vi "Example Before.vi"() -> ()   [LabVIEW 2019, in "LSS.lvlib"]
doc: "This example demonstrates how a user can save time developing user interfaces using LSS by showing how a simple application that uses property nodes to change style at runtime can be transitioned to using LSS. The \"Example Before.vi\" contains one way the code could have been written using arrays of property nodes. The \"Example After.vi\" is a functionally equivalent piece of code that uses LSS instead. Example After.vi uses no property nodes or manually created references to perform the exact same operations."
uses:
  LSS.lvlib
  SubVIs/Example SubVIs/Before SubVIs/Themes.ctl
  SubVIs/Example SubVIs/Before UI References.ctl
panel:
  out "mode":T1
  in  "Dialog":bool
  in  "Normal":bool
  in  "Small":bool
  in  "Slide 2":dbl(slide) scale=0.0..10.0
  out "Stat2":dbl
  out "Stat1":dbl
  out "Pressure":dbl
  out "Time":dbl
  in  "Slide":dbl(slide) scale=0.0..10.0
  in  "THEME2":bool
  in  "THEME1":bool
  in  "COMPANY":bool
  out "Mars":picture
  in  "SPACE":bool
  out "Map":picture
  out "Vortex":picture
  out "Chart 3":dbl(graph)
  out "Chart 2":dbl(graph)
  out "Chart1":dbl(graph)
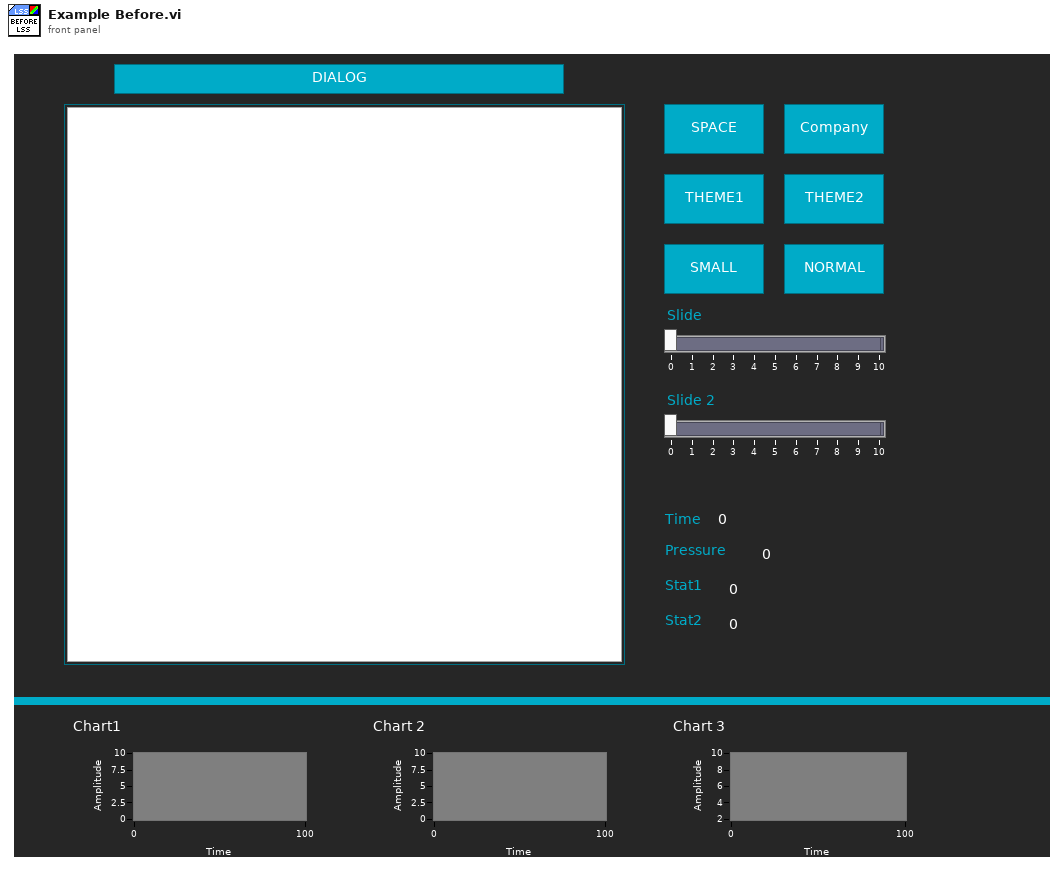
[diagram p1: front panel]
types:
  T1 = typedef "LSS.lvlib/Themes.ctl" = enum16{"SPACE", "COMPANY", "THEME1", "THEME2"}
  T2 = typedef "LSS.lvlib/Before UI References.ctl" = cluster{"Panes":refnum<vi>[], "Splitter":refnum<vi>, "Mars Picture":refnum<vi>, "Buttons":refnum<vi>[], "Numerics":refnum<vi>[], "Graphs":refnum<vi>[], "Slides":refnum<vi>[], "This VI":refnum<vi>, "Vortex":refnum<vi>, "Map":refnum<vi>}
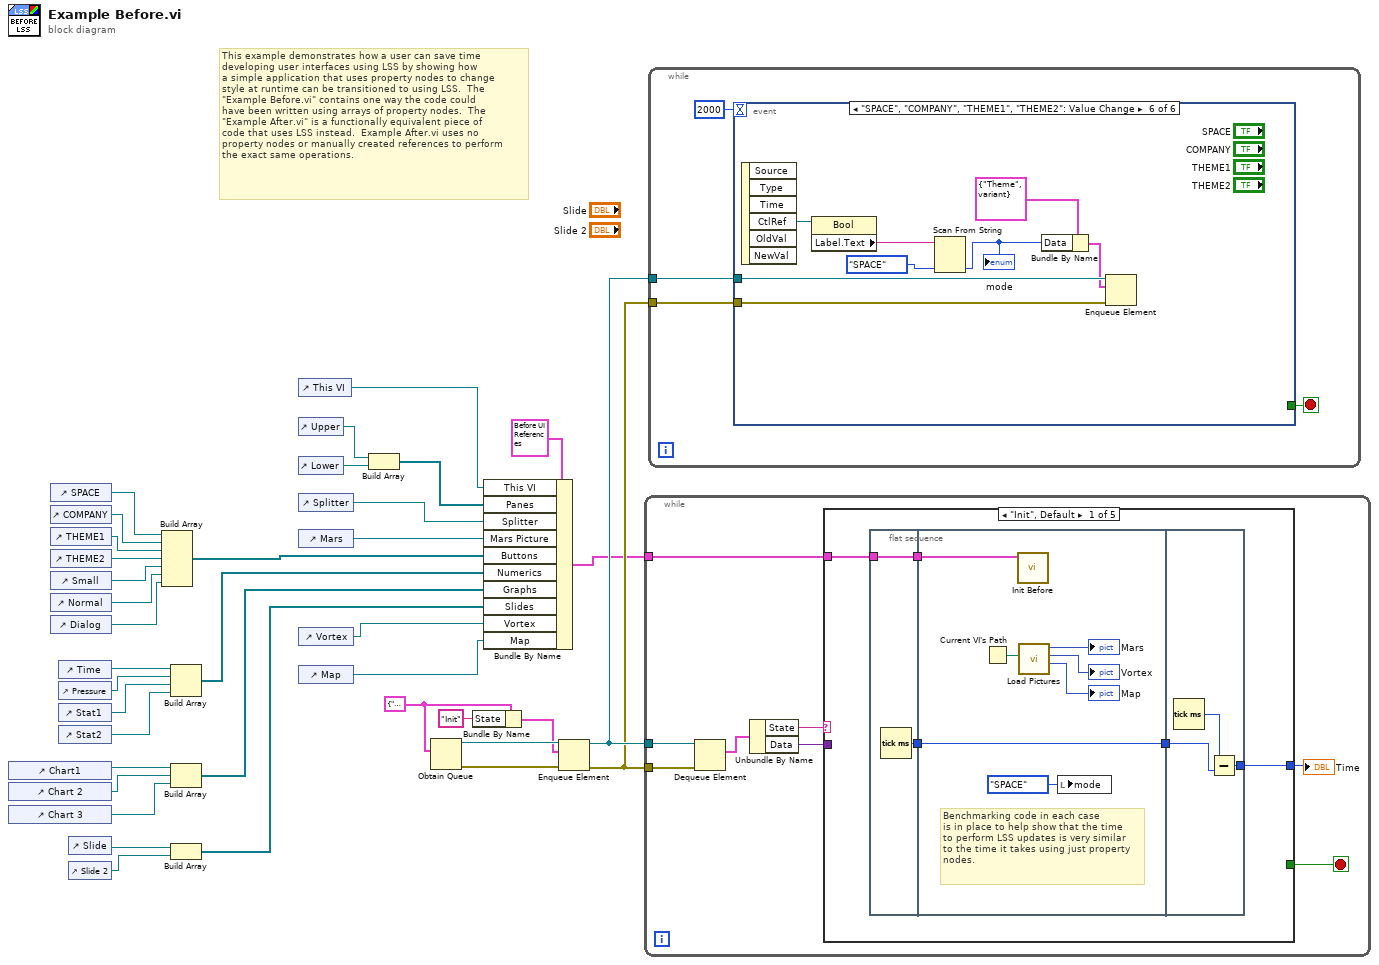
[diagram p0: block diagram]
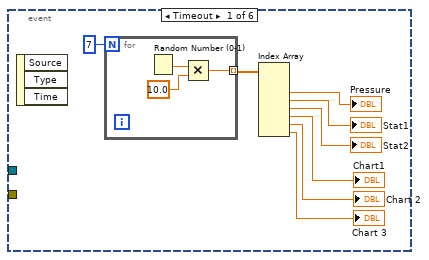
[diagram p2: hidden frame]
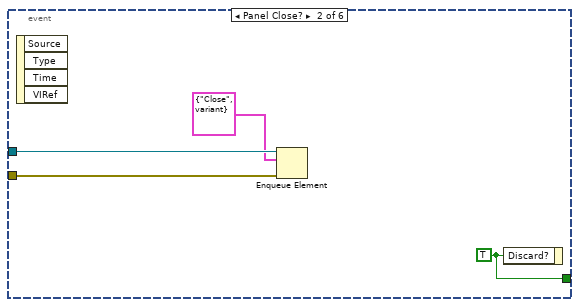
[diagram p3: hidden frame]
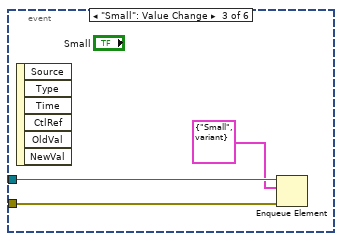
[diagram p4: hidden frame]
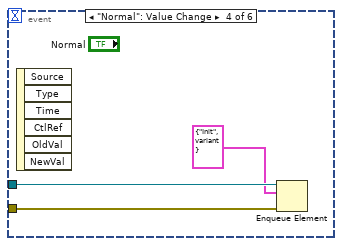
[diagram p5: hidden frame]
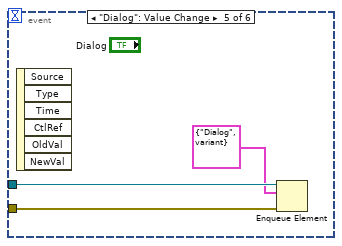
[diagram p6: hidden frame]
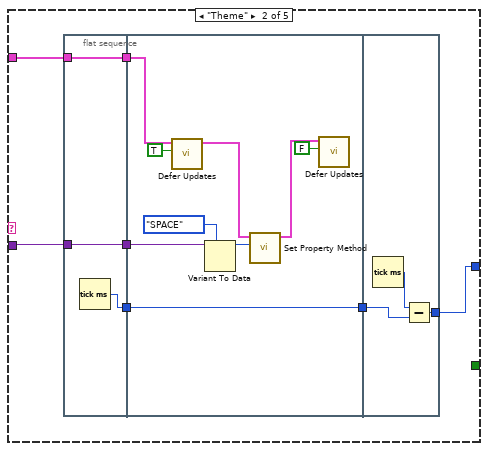
[diagram p7: hidden frame]
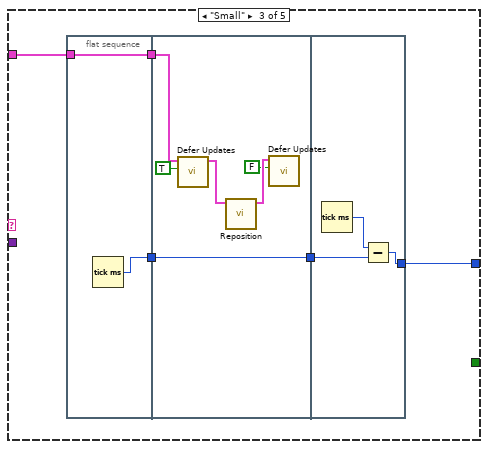
[diagram p8: hidden frame]
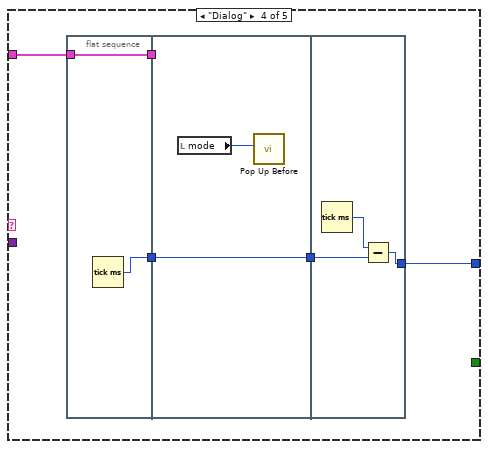
[diagram p9: hidden frame]
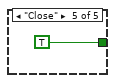
[diagram p10: hidden frame]
diagram:
  w35 = cluster{"State":string, "Data":variant} {"State"="", "Data"=variant}
  # "This example demonstrates how a user can save time\ndeveloping user interfaces using LSS by showing how\na simple application that uses property nodes to change\nstyle at runtime can be transitioned to using LSS.  The\n\"Example Before.vi\" contains one way the code could\nhave been written using arrays of property nodes.  The\n\"Example After.vi\" is a functionally equivalent piece of\ncode that uses LSS instead.  Example After.vi uses no\nproperty nodes or manually created references to perform\nthe exact same operations."
  n1 = control-ref of="Chart1"() -> (w14:refnum<vi>)
  n2 = control-ref of="Chart 2"() -> (w13:refnum<vi>)
  n3 = control-ref of="Chart 3"() -> (w12:refnum<vi>)
  n4 = control-ref of="SPACE"() -> (w20:refnum<vi>)
  n5 = control-ref of="COMPANY"() -> (w21:refnum<vi>)
  n6 = control-ref of="THEME1"() -> (w22:refnum<vi>)
  n7 = control-ref of="THEME2"() -> (w23:refnum<vi>)
  n8 = control-ref of="Small"() -> (w6:refnum<vi>)
  n9 = control-ref of="Normal"() -> (w5:refnum<vi>)
  n10 = control-ref of="Dialog"() -> (w3:refnum<vi>)
  n11 = control-ref of="Time"() -> (w18:refnum<vi>)
  n12 = control-ref of="Pressure"() -> (w17:refnum<vi>)
  n13 = control-ref of="Stat1"() -> (w16:refnum<vi>)
  n14 = control-ref of="Stat2"() -> (w15:refnum<vi>)
  n15 = control-ref of="Slide"() -> (w11:refnum<vi>)
  n16 = control-ref of="Slide 2"() -> (w10:refnum<vi>)
  n17 = Build Array(w20, w21, w22, w23, w6, w5, w3) -> (w19:refnum<vi>[])
  n18 = Build Array(w18, w17, w16, w15) -> (w9:refnum<vi>[])
  n19 = Build Array(w14, w13, w12) -> (w8:refnum<vi>[])
  n20 = Build Array(w11, w10) -> (w7:refnum<vi>[])
  n21 = control-ref of="This VI"() -> (w4:refnum<vi>)
  n22 = control-ref of="Upper"() -> (w30:refnum<vi>)
  n23 = control-ref of="Lower"() -> (w29:refnum<vi>)
  n24 = control-ref of="Splitter"() -> (w26:refnum<vi>)
  n25 = control-ref of="Mars"() -> (w25:refnum<vi>)
  n26 = control-ref of="Vortex"() -> (w2:refnum<vi>)
  n27 = control-ref of="Map"() -> (w1:refnum<vi>)
  n28 = Build Array(w30, w29) -> (w27:refnum<vi>[])
  n29 = Obtain Queue(element data type=w35) -> (queue out=w37:refnum<queue>, error out=w36:errorcluster)  [unwired: 4 in, 1 out]
  n30 = Bundle By Name(cluster=w35, "State"="Init") -> (w33:cluster{"State":string, "Data":variant})
  n31 = Bundle By Name(cluster=T2 {"Panes"=[], "Splitter"=refnum, "Mars Picture"=refnum, "Buttons"=[], "Numerics"=[], "Graphs"=[], "Slides"=[], "This VI"=refnum, "Vortex"=refnum, "Map"=refnum}, "This VI"=w4, "Panes"=w27, "Splitter"=w26, "Mars Picture"=w25, "Buttons"=w19, "Numerics"=w9, "Graphs"=w8, "Slides"=w7, "Vortex"=w2, "Map"=w1) -> (w24:T2)
  n32 = Enqueue Element(queue=w37, element=w33, error in (no error)=w36) -> (queue out=w32:refnum<queue>, error out=w31:errorcluster)  [unwired: 1 in, 1 out]
  n33 = while {
    tunnel: w32 -> [w45]
    tunnel: w31 -> [w44]
    tunnel: w24 -> [w39]
    stop <- w40 stop-if-true
    n34 = Dequeue Element(queue=w45, error in (no error)=w44) -> (element=w43:cluster{"State":string, "Data":variant})  [unwired: 1 in, 3 out]
    n35 = Unbundle By Name(w43) -> ("State"=w42:string, "Data"=w41:variant)
    n36 = case shown="\"Init\", Default" w42 {
      tunnel: w41 -> [_ w69 _ _ _]
      tunnel: [_ _ _ _ TRUE] -> w40
      tunnel: w39 -> [w50 w68 w89 w105 _]
      tunnel: [w46 w63 w85 w101 _] -> w38
      frame "Init", Default {
        n37 = flat-sequence {
          tunnel: w50 -> [w52]
          tunnel: [w52] -> w49
          tunnel: [w51] -> w48
          tunnel: w49 -> [w58]
          tunnel: w48 -> [w55]
          tunnel: [w55] -> w47
          tunnel: w47 -> [w62]
          tunnel: [w60] -> w46
          frame #0 {
            n38 = Tick Count (ms)() -> (millisecond timer value=w51:u32)
          }
          frame #1 {
            # "Benchmarking code in each case\nis in place to help show that the time\nto perform LSS updates is very similar\nto the time it takes using just property\nnodes."
            n39 = Current VI's Path() -> (path=w53:path)
            n40 = call "Init Before.vi"("Cluster"=w58) -> ()  [unwired: 11 in]
            n41 = call "Load Pictures.vi"("Application Directory"=w53) -> ("Map"=→"Map":picture, "Vortex"=→"Vortex":picture, "Mars"=→"Mars":picture)  [unwired: 8 in]
            n42 = local write "mode"(Themes."SPACE" ("mode")) -> ()
          }
          frame #2 {
            n43 = Tick Count (ms)() -> (millisecond timer value=w61:u32)
            n44 = Subtract(x=w61, y=w62) -> (x-y=w60:u32)
          }
        }
      }
      frame "Theme" {
        n45 = flat-sequence {
          tunnel: w68 -> [w71]
          tunnel: w69 -> [w72]
          tunnel: [w72] -> w67
          tunnel: [w71] -> w66
          tunnel: [w70] -> w64
          tunnel: w67 -> [w81]
          tunnel: w66 -> [w77]
          tunnel: [w78] -> w65
          tunnel: w64 -> [w78]
          tunnel: w65 -> [w83]
          tunnel: [w82] -> w63
          frame #0 {
            n46 = Tick Count (ms)() -> (millisecond timer value=w70:u32)
          }
          frame #1 {
            n47 = call "Defer Updates.vi"("Defer Panel Updates"=TRUE, "Cluster"=w77) -> ("Cluster Out"=w75:T2)  [unwired: 8 in, 1 out]
            n48 = Variant To Data(type=Themes."SPACE" ("Theme Choice"), Variant=w81) -> (data=w79:T1)  [unwired: 1 in, 1 out]
            n49 = call "Set Property Method.vi"("Theme Choice"=w79, "Cluster"=w75) -> ("Cluster Out"=w74:T2)  [unwired: 9 in]
            n50 = call "Defer Updates.vi"("Defer Panel Updates"=FALSE, "Cluster"=w74) -> ()  [unwired: 8 in, 2 out]
          }
          frame #2 {
            n51 = Tick Count (ms)() -> (millisecond timer value=w84:u32)
            n52 = Subtract(x=w84, y=w83) -> (x-y=w82:u32)
          }
        }
      }
      frame "Small" {
        n53 = flat-sequence {
          tunnel: w89 -> [w91]
          tunnel: [w91] -> w88
          tunnel: [w90] -> w86
          tunnel: w88 -> [w96]
          tunnel: [w97] -> w87
          tunnel: w86 -> [w97]
          tunnel: w87 -> [w99]
          tunnel: [w98] -> w85
          frame #0 {
            n54 = Tick Count (ms)() -> (millisecond timer value=w90:u32)
          }
          frame #1 {
            n55 = call "Defer Updates.vi"("Defer Panel Updates"=TRUE, "Cluster"=w96) -> ("Cluster Out"=w95:T2)  [unwired: 8 in, 1 out]
            n56 = call "Reposition.vi"("Cluster"=w95) -> ("Cluster Out"=w94:T2)  [unwired: 10 in]
            n57 = call "Defer Updates.vi"("Defer Panel Updates"=FALSE, "Cluster"=w94) -> ()  [unwired: 8 in, 2 out]
          }
          frame #2 {
            n58 = Tick Count (ms)() -> (millisecond timer value=w100:u32)
            n59 = Subtract(x=w100, y=w99) -> (x-y=w98:u32)
          }
        }
      }
      frame "Dialog" {
        n60 = flat-sequence {
          tunnel: w105 -> [w107]
          tunnel: [w107] -> w104
          tunnel: [w106] -> w102
          tunnel: w104 -> [_]
          tunnel: [w109] -> w103
          tunnel: w102 -> [w109]
          tunnel: w103 -> [w111]
          tunnel: [w110] -> w101
          frame #0 {
            n61 = Tick Count (ms)() -> (millisecond timer value=w106:u32)
          }
          frame #1 {
            n62 = local read "mode"() -> (w108:T1)
            n63 = call "Pop Up Before.vi"("mode"=w108) -> ()  [unwired: 11 in]
          }
          frame #2 {
            n64 = Tick Count (ms)() -> (millisecond timer value=w112:u32)
            n65 = Subtract(x=w112, y=w111) -> (x-y=w110:u32)
          }
        }
      }
      frame "Close" {
      }
    }
    "Time" <- w38
  }
  n66 = while {
    tunnel: w32 -> [w117]
    tunnel: w31 -> [w116]
    stop <- w115 stop-if-true
    n67 = event shown="[5] \"SPACE\", \"COMPANY\", \"THEME1\", \"THEME2\": Value Change" {
      selector: _ -> [_ _ _ _ _ _]
      dyn-events: _ -> [_ _ _ _ _ _]
      timeout: 2000 -> [_ _ _ _ _ _]
      tunnel: w117 -> [_ w131 w135 w138 w141 w149]
      tunnel: w116 -> [_ w130 w134 w137 w140 w148]
      tunnel: [_ w132 _ _ _ _] -> w115
      event Timeout {
        n68 = event-data() -> ()  [unwired: 1 in, 3 out]
        n69 = for {
          N: 7 -> [_]
          tunnel: [w126] -> w124 mode=indexing
          n70 = Random Number (0-1)() -> (number: 0 to 1=w128:dbl)
          n71 = Multiply(x=w128, y=10.0) -> (x*y=w126:dbl)
        }
        n72 = Index Array(array=w124) -> (element #2=→"Pressure":dbl, element #3=→"Stat1":dbl, element #4=→"Stat2":dbl, element #5=→"Chart1":dbl, element #6=→"Chart 2":dbl, element #7=→"Chart 3":dbl)  [unwired: 7 in, 1 out]
      }
      event Panel Close? {
        w132 = TRUE ("Discard?")
        n73 = event-data() -> ()  [unwired: 1 in, 4 out]
        n74 = Enqueue Element(queue=w131, element=cluster{"State":string, "Data":variant} {"State"="Close", "Data"=variant}, error in (no error)=w130) -> ()  [unwired: 1 in, 3 out]
        n75 = event-data("Discard?"=w132) -> ()  [unwired: 1 in, 1 out]
      }
      event "Small": Value Change {
        n76 = event-data() -> ()  [unwired: 1 in, 6 out]
        n77 = Enqueue Element(queue=w135, element=cluster{"State":string, "Data":variant} {"State"="Small", "Data"=variant}, error in (no error)=w134) -> ()  [unwired: 1 in, 3 out]
      }
      event "Normal": Value Change {
        n78 = event-data() -> ()  [unwired: 1 in, 6 out]
        n79 = Enqueue Element(queue=w138, element=cluster{"State":string, "Data":variant} {"State"="Init", "Data"=variant}, error in (no error)=w137) -> ()  [unwired: 1 in, 3 out]
      }
      event "Dialog": Value Change {
        n80 = event-data() -> ()  [unwired: 1 in, 6 out]
        n81 = Enqueue Element(queue=w141, element=cluster{"State":string, "Data":variant} {"State"="Dialog", "Data"=variant}, error in (no error)=w140) -> ()  [unwired: 1 in, 3 out]
      }
      event "SPACE", "COMPANY", "THEME1", "THEME2": Value Change {
        n82 = event-data() -> ("CtlRef"=w145:refnum<vi>)  [unwired: 1 in, 5 out]
        n83 = property class="Bool"(reference=w145) -> ("Label.Text"=w144:string)  [unwired: 1 in, 2 out]
        n84 = Scan From String(input string=w144, default 1=Themes."SPACE" ("Theme Choice")) -> (output 1=w143:T1)  [unwired: 3 in, 3 out]
        "mode" <- w143
        n85 = Bundle By Name(cluster=cluster{"State":string, "Data":variant} {"State"="Theme", "Data"=variant} ("element"), "Data"=w143) -> (w146:cluster{"State":string, "Data":variant})
        n86 = Enqueue Element(queue=w149, element=w146, error in (no error)=w148) -> ()  [unwired: 1 in, 3 out]
      }
    }
  }
